vi "SLSC Create Hierarchy Parameters.vi"(8 "error in (no error)":errorcluster, 10 "RevA?":bool, 11 "Item Ref in":T1 format="%.0x") -> (0 "error out":errorcluster, 3 "Item Ref out":T1 format="%.0x")   [LabVIEW 2015, in "SLSC-12201 DIO System Explorer.lvlib"]
uses:
  SLSC-12201 DIO System Explorer.lvlib
  <vilib>/NI Veristand/Custom Device API/Custom Device Item Ref.ctl
  Shared/Constants.vi
  <vilib>/NI Veristand/Custom Device API/Set Item Property (String).vi
  <vilib>/NI Veristand/Custom Device API/Custom Device API.lvlib
  Shared/SLSC-12201 DIO Shared.lvlib
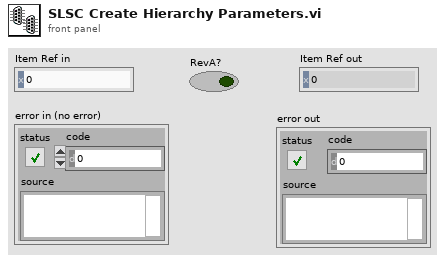
[diagram p1: front panel]
types:
  T1 = typedef "Custom Device API.lvlib/Custom Device Item Ref.ctl" = u64
  T2 = typedef "SLSC-12201 DIO System Explorer.lvlib/SLSC Channel Information.ctl" = cluster{"Channel Name":string, "SLSC Name":string, "Configuration":T3, "Enum Names":string[], "Enum Values":i32[]}
  T3 = typedef "Custom Device API.lvlib/Custom Device Channel.ctl" = cluster{"Type":T4, "Units":string, "Default Value":dbl, "Faultable":bool, "Scalable":bool}
  T4 = typedef "Custom Device API.lvlib/Custom Device Channel Type.ctl" = enum16{"Input", "Output"}
  T5 = cluster{"Channel Name":string, "SLSC Name":string, "Channel":T3, "Enum Names":string[], "Enum Values":i32[]}[]
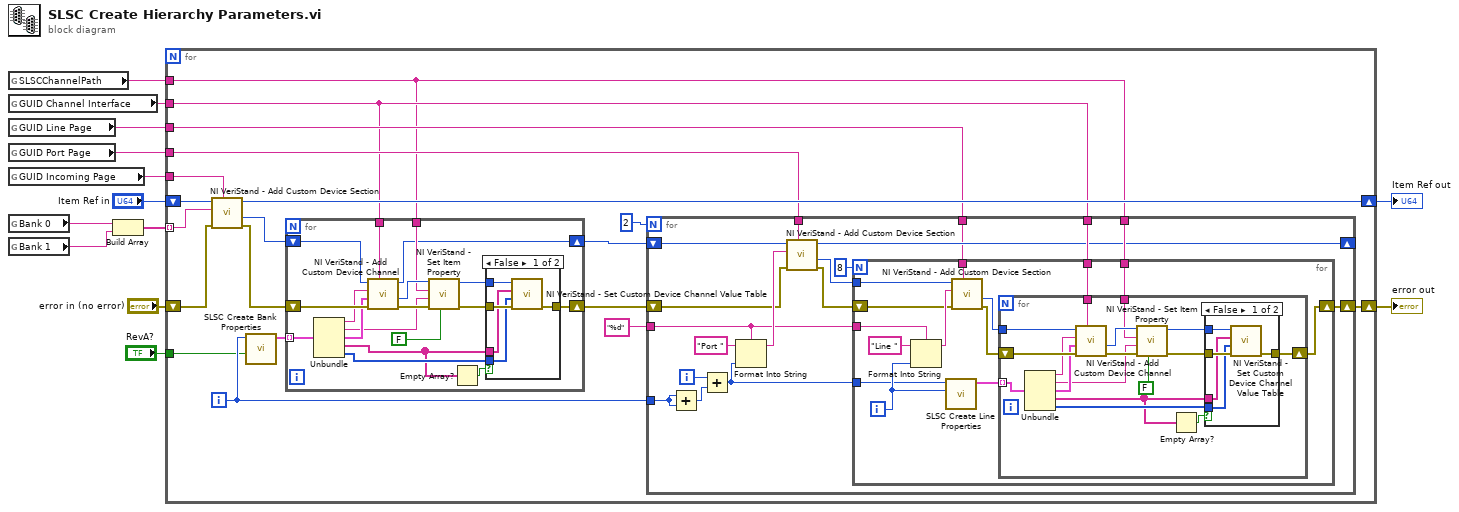
[diagram p0: block diagram]
diagram:
  n1 = global read "Constants.vi" "SLSCChannelPath"() -> (w3:string)
  n2 = global read "Constants.vi" "GUID Channel Interface"() -> (w4:string)
  n3 = global read "Constants.vi" "GUID Line Page"() -> (w6:string)
  n4 = global read "Constants.vi" "GUID Port Page"() -> (w5:string)
  n5 = global read "Constants.vi" "GUID Incoming Page"() -> (w2:string)
  n6 = global read "Constants.vi" "Bank 0"() -> (w11:string)
  n7 = global read "Constants.vi" "Bank 1"() -> (w12:string)
  n8 = Build Array(w11, w12) -> (w13:string[])
  n9 = for {
    shift-right: [w28] -> w9
    shift-left: "Item Ref in" -> [w32]
    shift-right: [w16] -> w10
    shift-left: "error in (no error)" -> [w31]
    tunnel: w13 -> [w27] mode=indexing
    tunnel: w6 -> [w25]
    tunnel: w5 -> [w24]
    tunnel: w4 -> [w23]
    tunnel: w3 -> [w22]
    tunnel: w2 -> [w21]
    tunnel: "RevA?" -> [w14]
    i -> [w26]
    n10 = call <vilib>:"NI VeriStand - Add Custom Device Section.vi"("GUID (Default Section)"=w21, "error in (no error)"=w31, "Section Name"=w27, "Parent Ref in"=w32) -> ("error out"=w17:errorcluster, "Section Ptr"=w20:T1, "Parent Ref out"=w28:T1)  [unwired: 4 in, 1 out]
    n11 = call "SLSC Create Bank Properties.vi"("RevA?"=w14, "Bank Number"=w26) -> ("Outgoing configuration"=w30:T2[])  [unwired: 8 in, 1 out]
    n12 = for {
      shift-right: [w91] -> w18
      shift-left: w17 -> [w102]
      tunnel: w22 -> [w103]
      tunnel: w23 -> [w95]
      tunnel: w30 -> [w101] mode=indexing
      shift-right: [w97] -> w19
      shift-left: w20 -> [w96]
      n13 = Unbundle(w101) -> ("Channel Name"=w100:string, "SLSC Name"=w98:string, "Configuration"=w99:T3, "Enum Names"=w89:string[], "Enum Values"=w90:i32[])
      n14 = call <vilib>:"NI VeriStand - Add Custom Device Channel.vi"("GUID (Default Channel)"=w95, "error in (no error)"=w102, "Channel"=w99, "Channel Name"=w100, "Parent Ref in"=w96) -> ("error out"=w104:errorcluster, "Channel Ref"=w105:T1, "Parent Ref out"=w97:T1)  [unwired: 3 in, 1 out]
      n15 = call-poly <vilib>:"NI VeriStand - Set Item Property.vi"("Binary String (T)"=FALSE, "error in (no error)"=w104, "Value"=w98, "Property Name"=w103, "Item Ref in"=w105) -> ("error out"=w92:errorcluster, "Item Ref out"=w93:T1)  [unwired: 4 in, 1 out]
      n16 = Empty Array?(array=w89) -> (empty?=w88:bool)
      n17 = case shown="False" w88 {
        tunnel: w93 -> [w110 _]
        tunnel: w92 -> [w109 w111]
        tunnel: [w108 w111] -> w91
        tunnel: w90 -> [w107 _]
        tunnel: w89 -> [w106 _]
        frame False {
          n18 = call <vilib>:"NI VeriStand - Set Custom Device Channel Value Table.vi"("error in (no error)"=w109, "Values"=w107, "Names"=w106, "Channel Ref in"=w110) -> ("error out"=w108:errorcluster)  [unwired: 6 in, 1 out]
        }
        frame True {
        }
      }
    }
    n19 = for {
      N: 2 -> [_]
      tunnel: w22 -> [w49]
      tunnel: w23 -> [w48]
      shift-right: [w43] -> _
      shift-left: w19 -> [w50]
      tunnel: w24 -> [w42]
      tunnel: w25 -> [w41]
      tunnel: w26 -> [w37]
      shift-right: [w40] -> w16
      shift-left: w18 -> [w35]
      tunnel: "%d" ("format string") -> [w33]
      i -> [w38]
      n20 = Add(x=w37, y=w37) -> (x+y=w36:i32)
      n21 = Add(x=w38, y=w36) -> (x+y=w34:i32)
      n22 = Format Into String(format string=w33, initial string="Port ", w34) -> (resulting string=w45:string)  [unwired: 1 in, 1 out]
      n23 = call <vilib>:"NI VeriStand - Add Custom Device Section.vi"("GUID (Default Section)"=w42, "error in (no error)"=w35, "Section Name"=w45, "Parent Ref in"=w50) -> ("error out"=w39:errorcluster, "Section Ptr"=w47:T1, "Parent Ref out"=w43:T1)  [unwired: 4 in, 1 out]
      n24 = for {
        N: 8 -> [_]
        tunnel: w49 -> [w63]
        tunnel: w48 -> [w62]
        tunnel: w47 -> [w59]
        tunnel: w34 -> [w57]
        tunnel: w41 -> [w55]
        shift-right: [w54] -> w40
        shift-left: w39 -> [w53]
        tunnel: w33 -> [w51]
        i -> [w58]
        n25 = Format Into String(format string=w51, initial string="Line ", w58) -> (resulting string=w61:string)  [unwired: 1 in, 1 out]
        n26 = call "SLSC Create Line Properties.vi"("Line Number"=w58, "Port Number"=w57) -> ("Outgoing configuration"=w64:T5)  [unwired: 9 in]
        n27 = call <vilib>:"NI VeriStand - Add Custom Device Section.vi"("GUID (Default Section)"=w55, "error in (no error)"=w53, "Section Name"=w61, "Parent Ref in"=w59) -> ("error out"=w52:errorcluster, "Section Ptr"=w56:T1)  [unwired: 4 in, 2 out]
        n28 = for {
          tunnel: w56 -> [w78]
          shift-right: [w68] -> w54
          shift-left: w52 -> [w77]
          tunnel: w63 -> [w79]
          tunnel: w62 -> [w72]
          tunnel: w64 -> [w76] mode=indexing
          n29 = Unbundle(w76) -> ("Channel Name"=w75:string, "SLSC Name"=w73:string, "Channel"=w74:T3, "Enum Names"=w66:string[], "Enum Values"=w67:i32[])
          n30 = call <vilib>:"NI VeriStand - Add Custom Device Channel.vi"("GUID (Default Channel)"=w72, "error in (no error)"=w77, "Channel"=w74, "Channel Name"=w75, "Parent Ref in"=w78) -> ("error out"=w80:errorcluster, "Channel Ref"=w81:T1)  [unwired: 3 in, 2 out]
          n31 = call-poly <vilib>:"NI VeriStand - Set Item Property.vi"("Binary String (T)"=FALSE, "error in (no error)"=w80, "Value"=w73, "Property Name"=w79, "Item Ref in"=w81) -> ("error out"=w69:errorcluster, "Item Ref out"=w65:T1)  [unwired: 4 in, 1 out]
          n32 = Empty Array?(array=w66) -> (empty?=w70:bool)
          n33 = case shown="False" w70 {
            tunnel: w65 -> [w86 _]
            tunnel: w69 -> [w85 w87]
            tunnel: [w84 w87] -> w68
            tunnel: w67 -> [w83 _]
            tunnel: w66 -> [w82 _]
            frame False {
              n34 = call <vilib>:"NI VeriStand - Set Custom Device Channel Value Table.vi"("error in (no error)"=w85, "Values"=w83, "Names"=w82, "Channel Ref in"=w86) -> ("error out"=w84:errorcluster)  [unwired: 6 in, 1 out]
            }
            frame True {
            }
          }
        }
      }
    }
  }
  "error out" <- w10
  "Item Ref out" <- w9
